vi "Аккумулятор 1.vi"(1 "Reset":bool, 2 "C":bool, 3 "d":T1) -> (0 "output":T2)   [LabVIEW 2017]
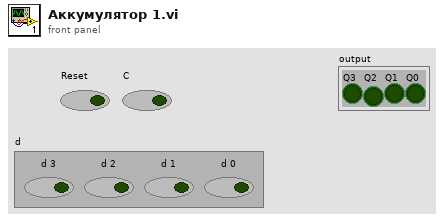
[diagram p1: front panel]
types:
  T1 = cluster{"d 3":bool, "d 2 ":bool, "d 1":bool, "d 0":bool}
  T2 = cluster{"Q3":bool, "Q2":bool, "Q1":bool, "Q0":bool}
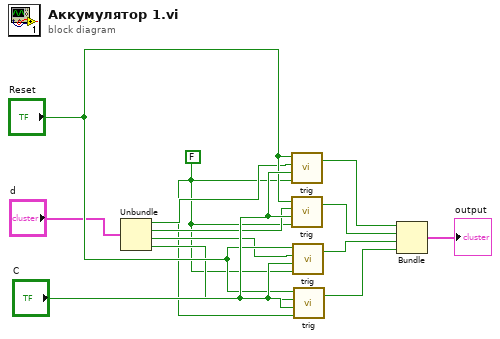
[diagram p0: block diagram]
diagram:
  w1 = FALSE
  n1 = Unbundle("d") -> ("d 3"=w2:bool, "d 2"=w3:bool, "d 1"=w4:bool, "d 0"=w5:bool)
  n2 = call "trig.vi"("s"=w1, "c"="C", "d"=w2, "r"="Reset") -> ("q"=w9:bool)  [unwired: 1 out]
  n3 = call "trig.vi"("s"=w1, "c"="C", "d"=w3, "r"="Reset") -> ("q"=w10:bool)  [unwired: 1 out]
  n4 = call "trig.vi"("s"=w1, "c"="C", "d"=w4, "r"="Reset") -> ("q"=w11:bool)  [unwired: 1 out]
  n5 = call "trig.vi"("s"=w1, "c"="C", "d"=w5, "r"="Reset") -> ("q"=w12:bool)  [unwired: 1 out]
  n6 = Bundle("q"=w9, "q"=w10, "q"=w11, "q"=w12) -> (→"output":cluster{"q":bool, "q":bool, "q":bool, "q":bool})  [unwired: 1 in]
